vi "MathSubsidaries1.vi"() -> ()   [LabVIEW 2020]
panel:
  out "sum":dbl
  out "result":dbl
  out "x-1":dbl
  out "x+y":dbl
  in  "y":dbl
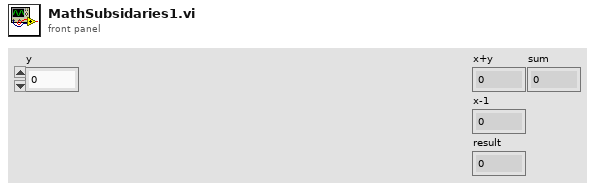
[diagram p1: front panel]
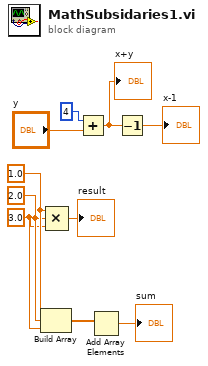
[diagram p0: block diagram]
diagram:
  w3 = 3.0 ("value")
  w4 = 2.0 ("value")
  w5 = 1.0 ("value")
  n1 = Build Array(w5, w4, w3) -> (w2:dbl[])
  n2 = Compound Arithmetic op=MULTIPLY(w5, w4, w3) -> (→"result":dbl)
  n3 = Add(x=4, y="y") -> (x+y=w8:dbl)
  "x+y" <- w8
  n4 = Add Array Elements(numeric array=w2) -> (sum=→"sum":dbl)
  n5 = Decrement(x=w8) -> (x-1=→"x-1":dbl)
